vi "Actor Core.vi"(8 "error in":errorcluster, 11 "Nested in":refnum<class "[MV] Key Certify.lvclass">) -> (0 "error out":errorcluster, 3 "Actor out":refnum<class "Actor.lvclass">)   [LabVIEW 2023, in "[MV] Key Certify.lvlib" / "[MV] Key Certify.lvclass"]
doc: "(<B>Filename</B>: Actor Framework.lvlib:Actor.lvclass:Actor Core.vi)\n\nReceives messages to the actor, reacts to them, and initiates any error handling that may shut the actor down.\n\nDescendant classes may override this VI to append parallel tasks for the actor to complete while it handles messages. Overrides use the Call Parent Method node."
uses:
  [MV] Key Certify.lvclass
  C:/Program Files (x86)/National Instruments/LabVIEW 2023/vi.lib/ActorFramework/Actor/Actor.lvclass
  <vilib>/ActorFramework/Actor/Actor.lvclass
  <vilib>/ActorFramework/Actor/Actor.lvclass/Actor.ctl
  <vilib>/ActorFramework/Message Enqueuer/Message Enqueuer.lvclass/Message Enqueuer.ctl
  [MV] Key Certify.lvclass/[MV] Key Certify.ctl
  <vilib>/ActorFramework/Message Enqueuer/Init from Existing Queue.vi
  <vilib>/ActorFramework/Message Enqueuer/Enqueue.vi
  [MV] Key Certify Messages/Event Active Msg/Event Active Msg.lvclass
  C:/Program Files (x86)/National Instruments/LabVIEW 2023/vi.lib/ActorFramework/Message/Message.lvclass
  <vilib>/ActorFramework/Stop Msg/Stop Msg.lvclass
  <vilib>/ActorFramework/Message Priority Queue/Priority Enqueue.vi
  <vilib>/ActorFramework/Message Enqueuer/Message Enqueuer.lvclass
panel:
  in  "active":bool
  in  "key":string caption="激活码"
  out "machine code":string caption="机器码"
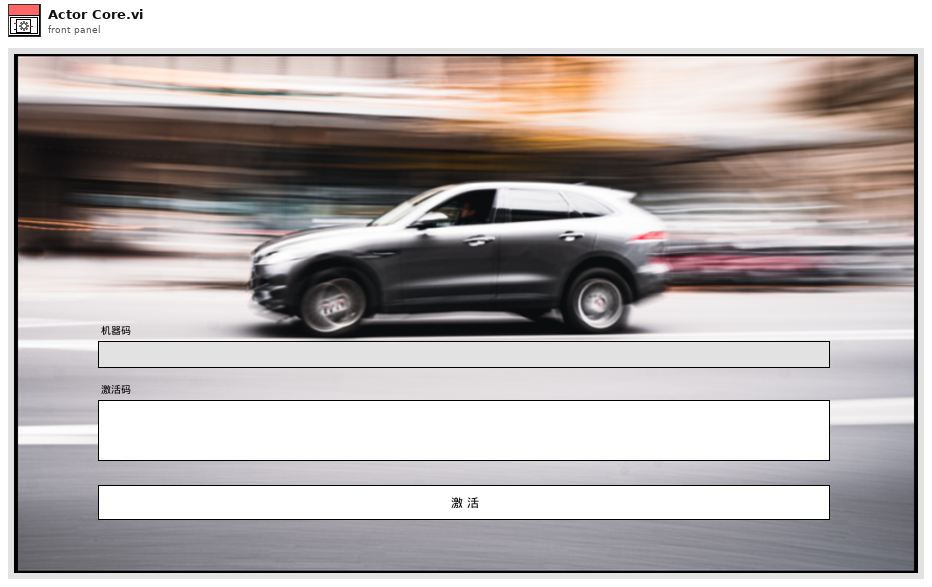
[diagram p1: front panel]
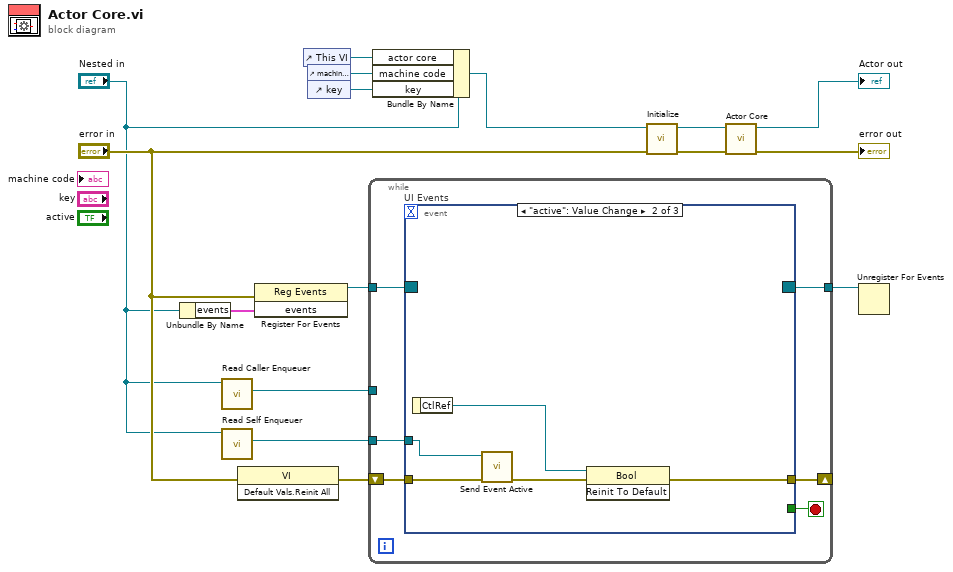
[diagram p0: block diagram]
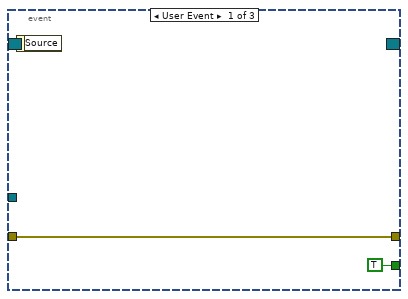
[diagram p2: hidden frame]
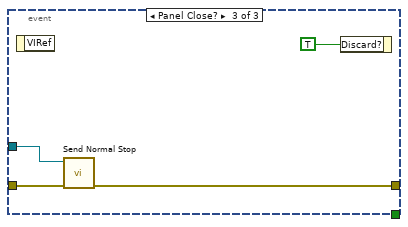
[diagram p3: hidden frame]
diagram:
  n1 = Unbundle By Name("Nested in") -> ("events"=w13:cluster{"stop":refnum<user-event>})
  n2 = call <vilib>:"Read Caller Enqueuer.vi"("Actor"="Nested in") -> ("Caller Enqueuer"=w10:refnum<class "Message Enqueuer.lvclass">)  [unwired: 10 in]
  n3 = call <vilib>:"Read Self Enqueuer.vi"("Actor"="Nested in") -> ("Self Enqueuer"=w11:refnum<class "Message Enqueuer.lvclass">)  [unwired: 10 in]
  n4 = invoke class="VI" method="Default Vals.Reinit All"(error in="error in") -> (error out=w9:errorcluster)  [unwired: 2 in, 2 out]
  n5 = register-events ("Main Register for Events")(error in="error in", w13) -> (reference out=w14:refnum<event-registration>)  [unwired: 1 in, 1 out]
  n6 = control-ref of="This VI"() -> (w1:refnum<vi>)
  n7 = control-ref of="machine code"() -> (w3:refnum<vi>)
  n8 = control-ref of="key"() -> (w2:refnum<vi>)
  n9 = while {
    tunnel: w14 -> [w22]
    tunnel: [w20] -> w12
    tunnel: w11 -> [w19]
    tunnel: w10 -> [_]
    shift-right: [w17] -> _
    shift-left: w9 -> [w18]
    stop <- w21 stop-if-true
    n10 = event "UI Events" shown="[1] \"active\": Value Change" {
      selector: w22 -> [_ _ _]
      dyn-events: [_ _ _] -> w20
      timeout: _ -> [_ _ _]
      tunnel: [TRUE _ _] -> w21
      tunnel: w19 -> [_ w28 w32]
      tunnel: w18 -> [w24 w29 w31]
      tunnel: [w24 w25 w30] -> w17
      event User Event {
        n11 = event-data() -> ()  [unwired: 1 in, 1 out]
      }
      event "active": Value Change {
        n12 = event-data() -> ("CtlRef"=w26:refnum<vi>)  [unwired: 1 in]
        n13 = call "Send Event Active.vi"("error in (no error)"=w29, "Message Enqueuer"=w28) -> ("error out"=w27:errorcluster)  [unwired: 8 in, 1 out]
        n14 = invoke class="Bool" method="Reinit To Default"(reference=w26, error in=w27) -> (error out=w25:errorcluster)  [unwired: 1 in, 2 out]
      }
      event Panel Close? {
        n15 = event-data() -> ()  [unwired: 1 in, 1 out]
        n16 = call <vilib>:"Send Normal Stop.vi"("error in (no error)"=w31, "Message Enqueuer"=w32) -> ("error out"=w30:errorcluster)  [unwired: 9 in]
        n17 = event-data("Discard?"=TRUE) -> ()  [unwired: 1 in, 1 out]
      }
    }
  }
  n18 = Bundle By Name(cluster="Nested in", "actor core"=w1, "machine code"=w3, "key"=w2) -> (w4:refnum<class "[MV] Key Certify.lvclass">)
  n19 = call "Initialize.vi"("error in (no error)"="error in", "View Template in"=w4) -> ("error out"=w8:errorcluster, "View Template out"=w7:refnum<class "[MV] Key Certify.lvclass">)  [unwired: 8 in]
  n20 = call-parent "Actor Core.vi"("error in"=w8, "Actor in"=w7) -> ("error out"=→"error out":errorcluster, "Actor out"=→"Actor out":refnum<class "Actor.lvclass">)  [unwired: 8 in]
  n21 = Unregister For Events(event registration refnum=w12) -> ()  [unwired: 1 in, 1 out]
